vi "Read Views User Event Ref.vi"(8 "error in (no error)":errorcluster, 11 "GUI Container in":refnum<class "GUI Container.lvclass">) -> (0 "error out":errorcluster, 2 "user event out":refnum<user-event>, 3 "GUI Container out":refnum<class "GUI Container.lvclass">)   [LabVIEW 2023, in "GUI Views.lvlib" / "GUI Container.lvclass"]
uses:
  GUI Container.lvclass
  GUI Container.lvclass/GUI Container.ctl
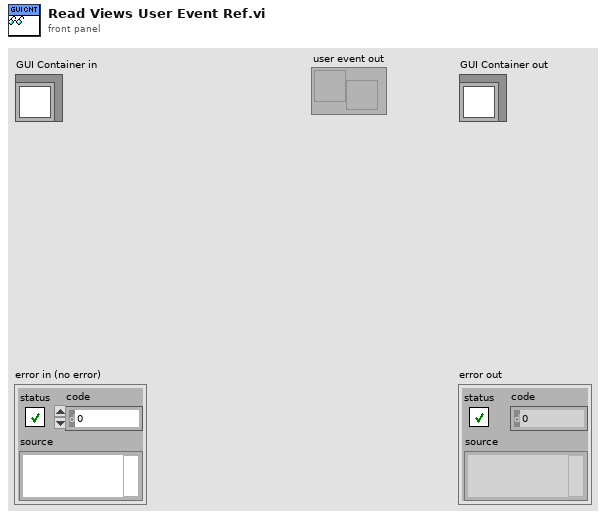
[diagram p1: front panel]
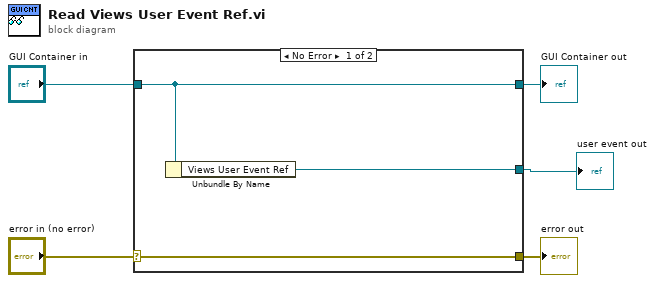
[diagram p0: block diagram]
diagram:
  n1 = case shown="No Error" "error in (no error)" {
    selector: "error in (no error)" -> [w8 w9]
    tunnel: [w8 w9] -> w4
    tunnel: [w7 w10] -> w2
    tunnel: "GUI Container in" -> [w7 w10]
    tunnel: [w6 _] -> w1
    frame No Error {
      n2 = Unbundle By Name(w7) -> ("Views User Event Ref"=w6:refnum<user-event>)
    }
    frame Error {
    }
  }
  "error out" <- w4
  "GUI Container out" <- w2
  "user event out" <- w1
